vi "Launcher.vi"   [LabVIEW 2019]
uses:
  TypeDef/SM_launcher.ctl
  <vilib>/ErrorRing/Error Ring.xnode
  Libraries/Server/Server.lvlib
types:
  T1 = typedef "SM_launcher.ctl" = enum16{"close", "start", "event"}
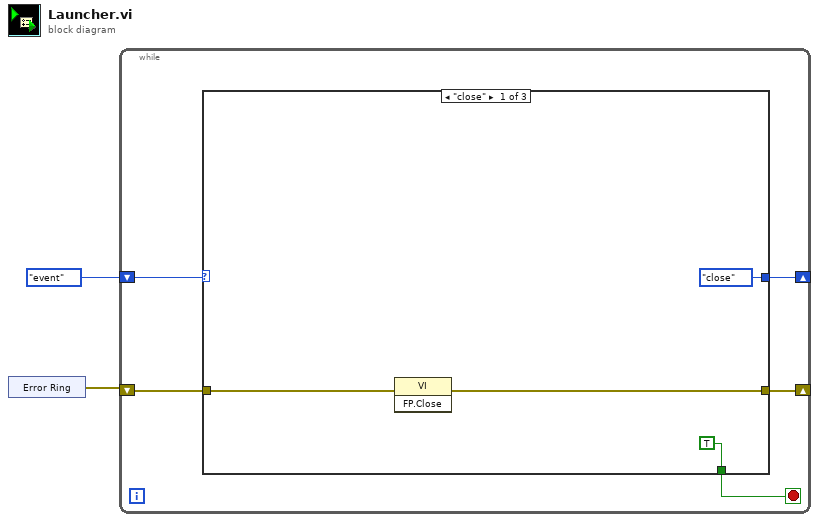
[diagram p0: block diagram]
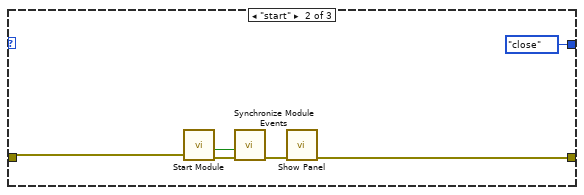
[diagram p2: hidden frame]
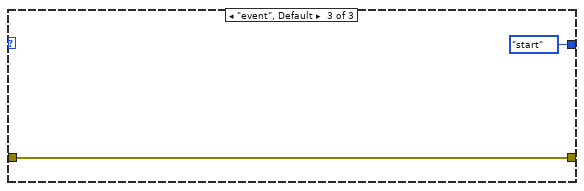
[diagram p3: hidden frame]
diagram:
  n1 = xnode "Error Ring"() -> ("error out"=w1:errorcluster)
  n2 = while {
    shift-right: [w5] -> _
    shift-left: SM_launcher."event" ("Enum") -> [w7]
    shift-right: [w4] -> _
    shift-left: w1 -> [w3]
    stop <- w6 stop-if-true
    n3 = case shown="\"close\"" w7 {
      tunnel: [TRUE _ _] -> w6
      tunnel: [SM_launcher."close" ("Enum") SM_launcher."close" ("Enum") SM_launcher."start" ("Enum")] -> w5
      tunnel: [w8 w13 w18] -> w4
      tunnel: w3 -> [w9 w12 w18]
      frame "close" {
        n4 = invoke class="VI" method="FP.Close"(error in=w9) -> (error out=w8:errorcluster)  [unwired: 2 in, 2 out]
      }
      frame "start" {
        n5 = call "Start Module.vi"("error in (no error)"=w12) -> ("error out"=w15:errorcluster, "Wait for Event Sync?"=w16:bool)  [unwired: 7 in, 2 out]
        n6 = call "Synchronize Module Events.vi"("error in (no error)"=w15, "Wait for Event Sync?"=w16) -> ("error out"=w14:errorcluster)  [unwired: 9 in]
        n7 = call "Show Panel.vi"("error in (no error)"=w14) -> ("error out"=w13:errorcluster)  [unwired: 10 in]
      }
      frame "event", Default {
      }
    }
  }
